vi "Get Endstop state.vi"(10 "ES array in":bool[](array[boolean]), 11 "Device model":string) -> (1 "ES array out":bool[](array[boolean]), 2 "ES2":bool, 3 "ES1":bool)   [LabVIEW 2020]
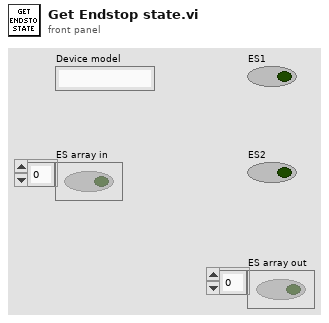
[diagram p1: front panel]
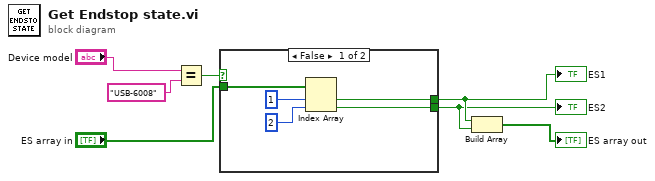
[diagram p0: block diagram]
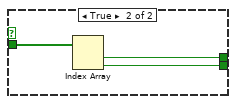
[diagram p2: hidden frame]
diagram:
  n1 = Equal?(x="Device model", y="USB-6008") -> (x = y?=w1:bool)
  n2 = case shown="False" w1 {
    tunnel: [w9 w15] -> w4
    tunnel: [w8 w14] -> w3
    tunnel: "ES array in" -> [w12 w13]
    frame False {
      n3 = Index Array(array=w12, index #1=1 ("index"), index #2=2 ("index")) -> (element #1=w9:bool, element #2=w8:bool)
    }
    frame True {
      n4 = Index Array(array=w13) -> (element #1=w15:bool, element #2=w14:bool)  [unwired: 2 in]
    }
  }
  "ES2" <- w3
  "ES1" <- w4
  n5 = Build Array(w4, w3) -> (→"ES array out":bool[])
